vi "SSL Detection Frame Simple Estimator Cameras VelCmd.vi"(0 "Side":enum16{"Esquerdo", "Direito"}(ring)=enum."Direito" caption="Enum", 1 "cameras array":dbl[](array[numeric]), 4 "max ball vel":dbl, 5 "Estimador":T6=enum."Nenhum", 6 "Team":enum16{"Azul", "Amarelo"}(ring) caption="Enum", 7 "Enable":bool=TRUE, 8 "Fps":dbl=40.0, 9 "grSim?":bool, 10 "Field":T1, 11 "Detection Frame":T2 {"robots_blue"."height" format="%+4.3f"; "robots_blue"."pixel_y" format="%+4.3f"; "robots_blue"."pixel_x" format="%+4.3f"; "robots_blue"."orientation" format="%+4.3f"; "robots_blue"."y" format="%+4.3f"; "robots_blue"."confidence" format="%4.3f"; "robots_blue"."x" format="%+4.3f"; "robots_yellow"."height" format="%+4.3f"; "robots_yellow"."pixel_y" format="%+4.3f"; "robots_yellow"."pixel_x" format="%+4.3f"; "robots_yellow"."orientation" format="%+4.3f"; "robots_yellow"."y" format="%+4.3f"; "robots_yellow"."confidence" format="%4.3f"; "robots_yellow"."x" format="%+4.3f"}) -> (2 "Field":T1, 3 "Detection Frame Out":T2 {"robots_blue"."height" format="%+4.3f"; "robots_blue"."pixel_y" format="%+4.3f"; "robots_blue"."pixel_x" format="%+4.3f"; "robots_blue"."orientation" format="%+4.3f"; "robots_blue"."y" format="%+4.3f"; "robots_blue"."confidence" format="%4.3f"; "robots_blue"."x" format="%+4.3f"; "robots_yellow"."height" format="%+4.3f"; "robots_yellow"."pixel_y" format="%+4.3f"; "robots_yellow"."pixel_x" format="%+4.3f"; "robots_yellow"."orientation" format="%+4.3f"; "robots_yellow"."y" format="%+4.3f"; "robots_yellow"."confidence" format="%4.3f"; "robots_yellow"."x" format="%+4.3f"})   [LabVIEW 2020]
uses:
  Controls/SSL Detection Frame.ctl
  Controls/SSL Detection Robot.ctl
  <vilib>/Analysis/Matrix/Datatypes/RealMatrix.ctl
  Controls/SSL Detection Ball.ctl
  Controls/Estimadores.ctl
  <vilib>/Analysis/Matrix/Numeric/Conversions/Array To Matrix - RA.vi
  <vilib>/Analysis/Matrix/NI_Matrix.lvlib
  <vilib>/ptbypt/NI_PtbyPt.lvlib
  Robot_class/FieldFIRASim.ctl
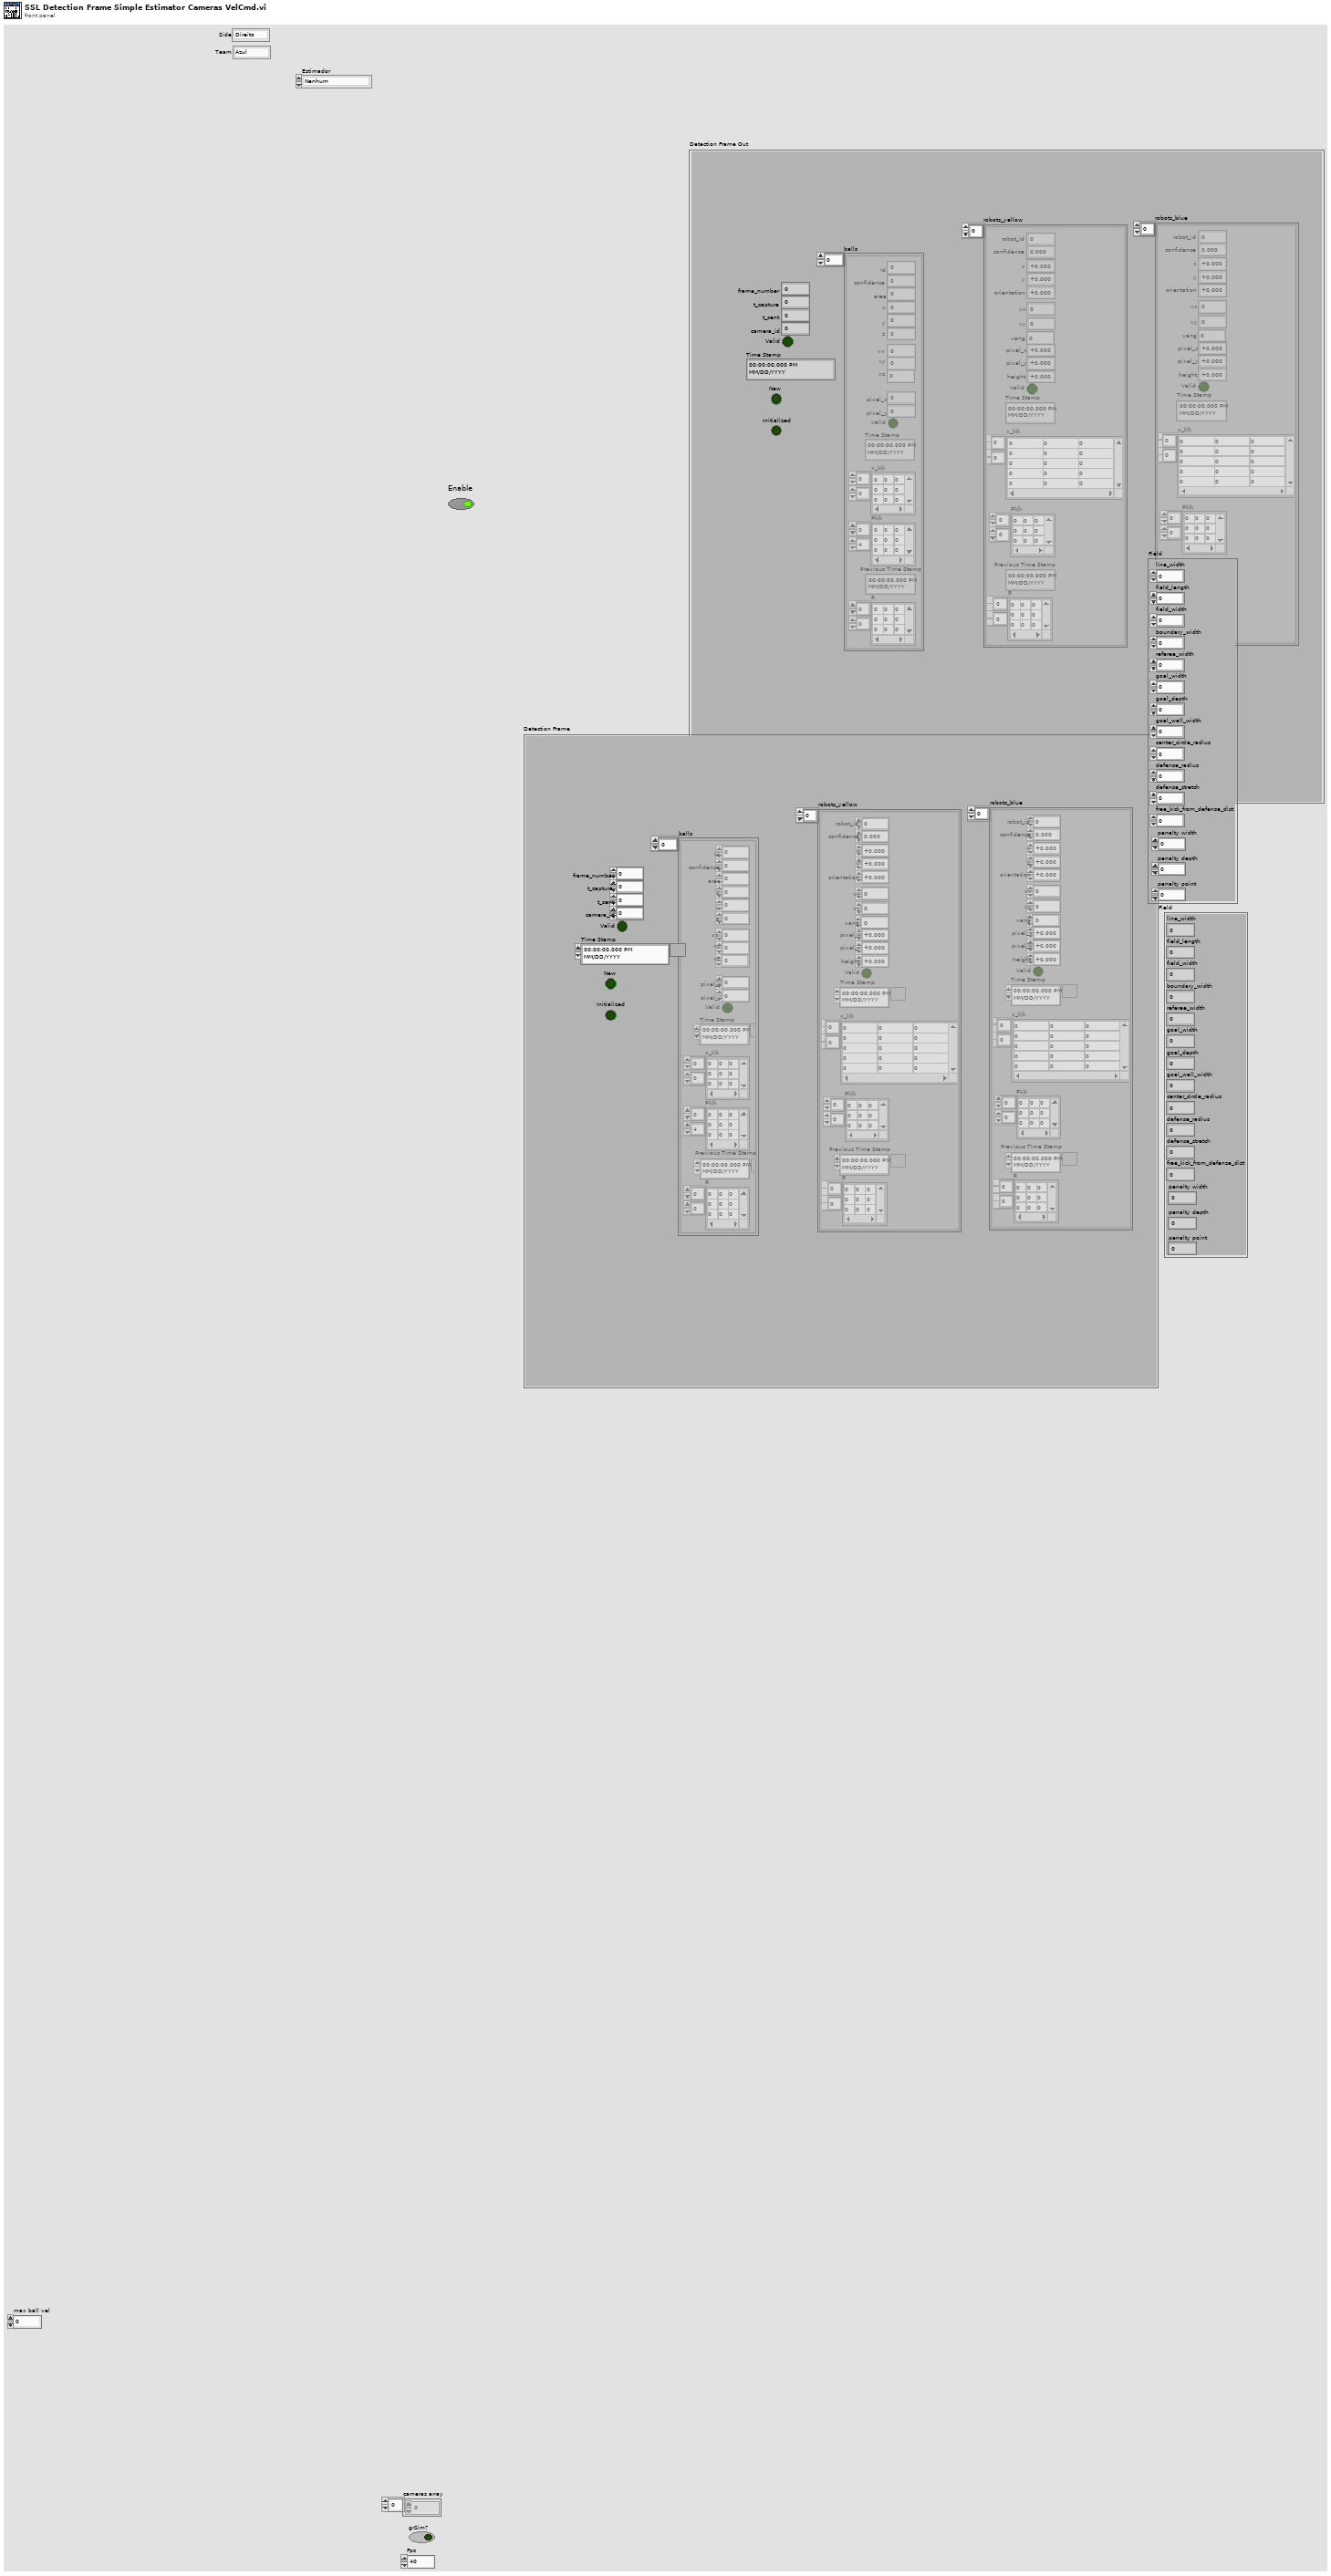
[diagram p1: front panel]
types:
  T1 = typedef "FieldFIRASim.ctl" = cluster{"line_width":u32, "field_length":u32, "field_width":u32, "boundary_width":u32, "referee_width":u32, "goal_width":u32, "goal_depth":u32, "goal_wall_width":u32, "center_circle_radius":u32, "defense_radius":u32, "defense_stretch":u32, "free_kick_from_defense_dist":u32, "penalty width":dbl, "penalty depth":dbl, "penalty point":dbl}
  T2 = typedef "SSL Detection Frame.ctl" = cluster{"frame_number":u32, "t_capture":dbl, "t_sent":dbl, "camera_id":u32, "robots_yellow":T3[], "robots_blue":T3[], "balls":T5[], "Valid":bool, "Time Stamp":timestamp, "New":bool, "Initialized":bool}
  T3 = typedef "SSL Detection Robot.ctl" = cluster{"x":sgl, "robot_id":u32, "confidence":sgl, "y":sgl, "orientation":sgl, "pixel_x":sgl, "pixel_y":sgl, "height":sgl, "Valid":bool, "Time Stamp":timestamp, "x_k|k":T4, "Pk|k":T4, "Previous Time Stamp":timestamp, "R":T4, "vx":dbl, "vy":dbl, "vang":dbl}
  T4 = typedef "NI_Matrix.lvlib/RealMatrix.ctl" = dbl[][]
  T5 = typedef "SSL Detection Ball.ctl" = cluster{"x":sgl, "area":u32, "confidence":sgl, "y":sgl, "z":sgl, "pixel_x":sgl, "pixel_y":sgl, "Valid":bool, "Time Stamp":timestamp, "x_k|k":T4, "Pk|k":T4, "Id":u32, "Previous Time Stamp":timestamp, "R":T4, " vx":sgl, "vy":dbl, "vz":dbl}
  T6 = typedef "Estimadores.ctl" = enum16{"4thDerivate", "2ndDerivate", "Nenhum", "Simples", "Kalman"}
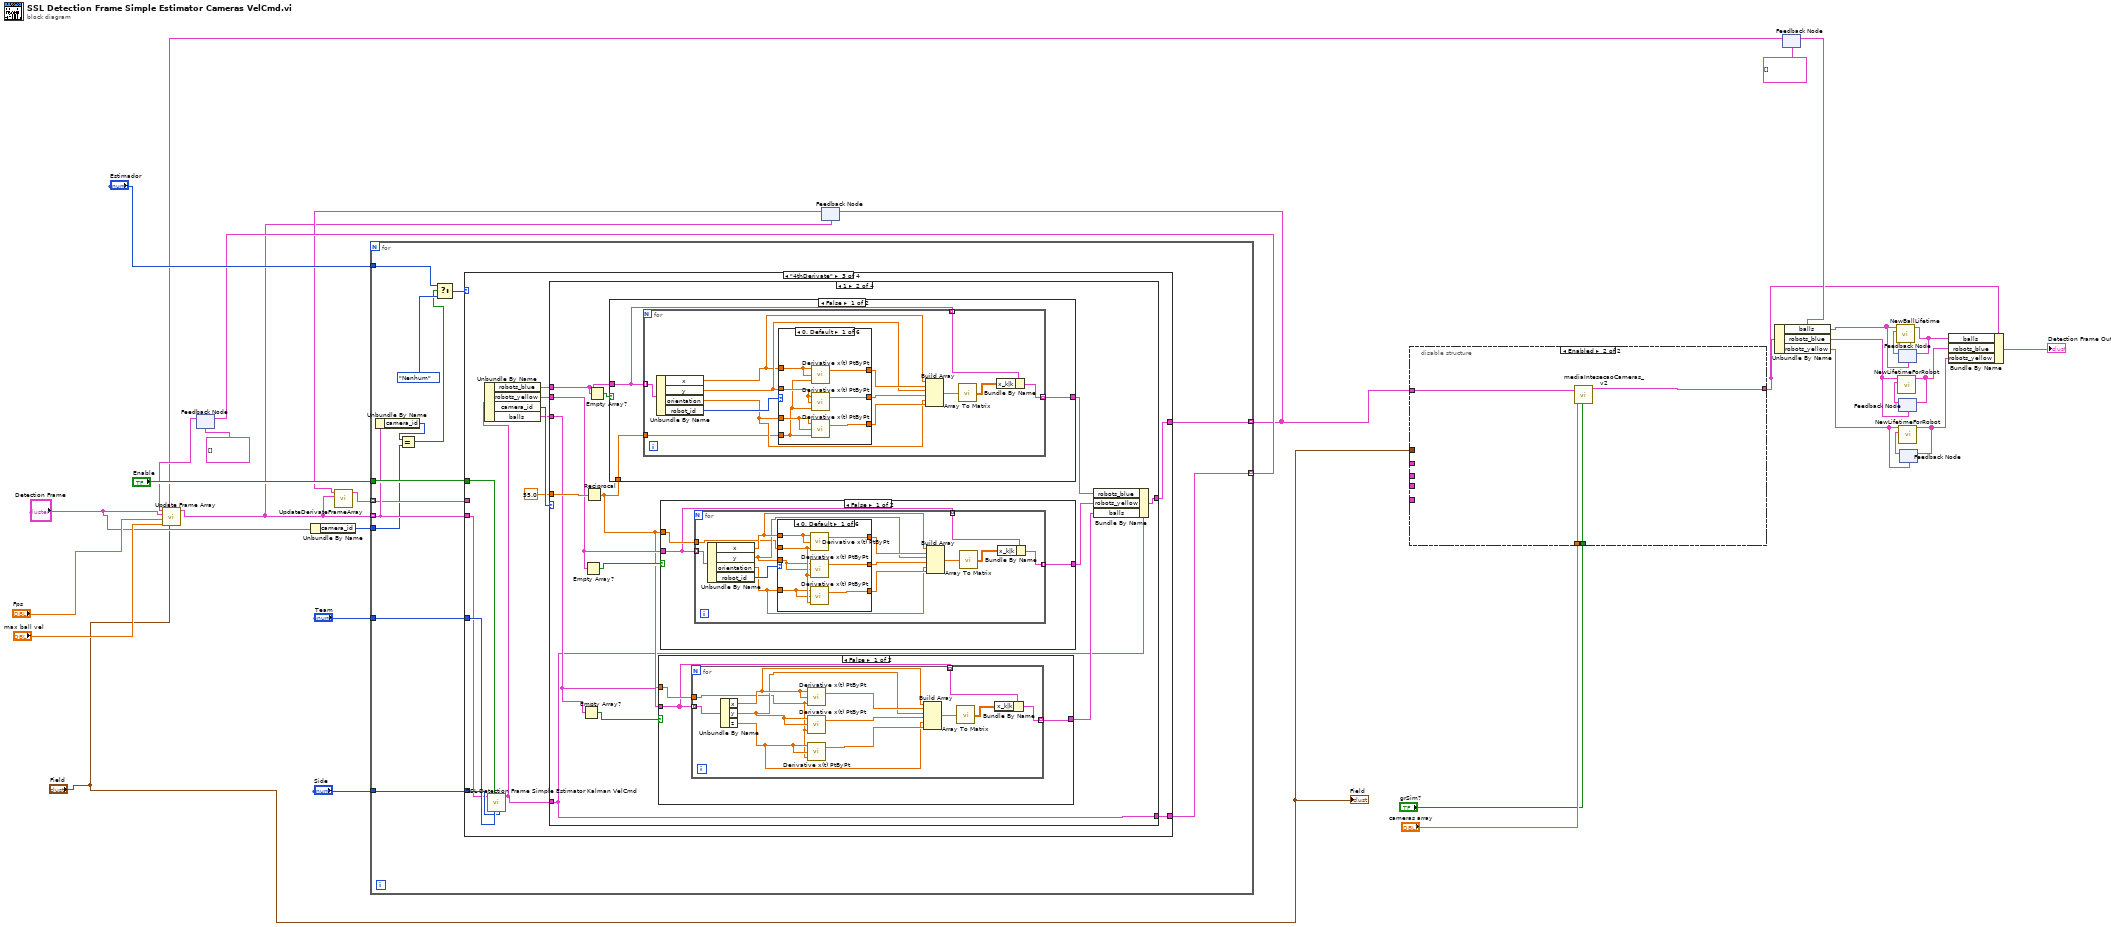
[diagram p0: block diagram]
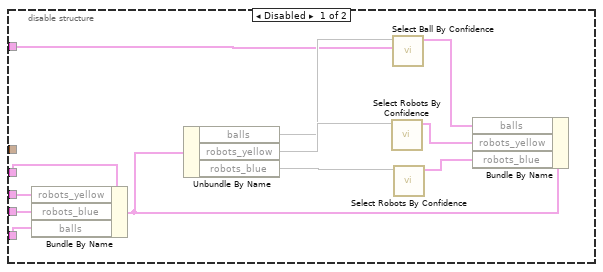
[diagram p2: hidden frame]
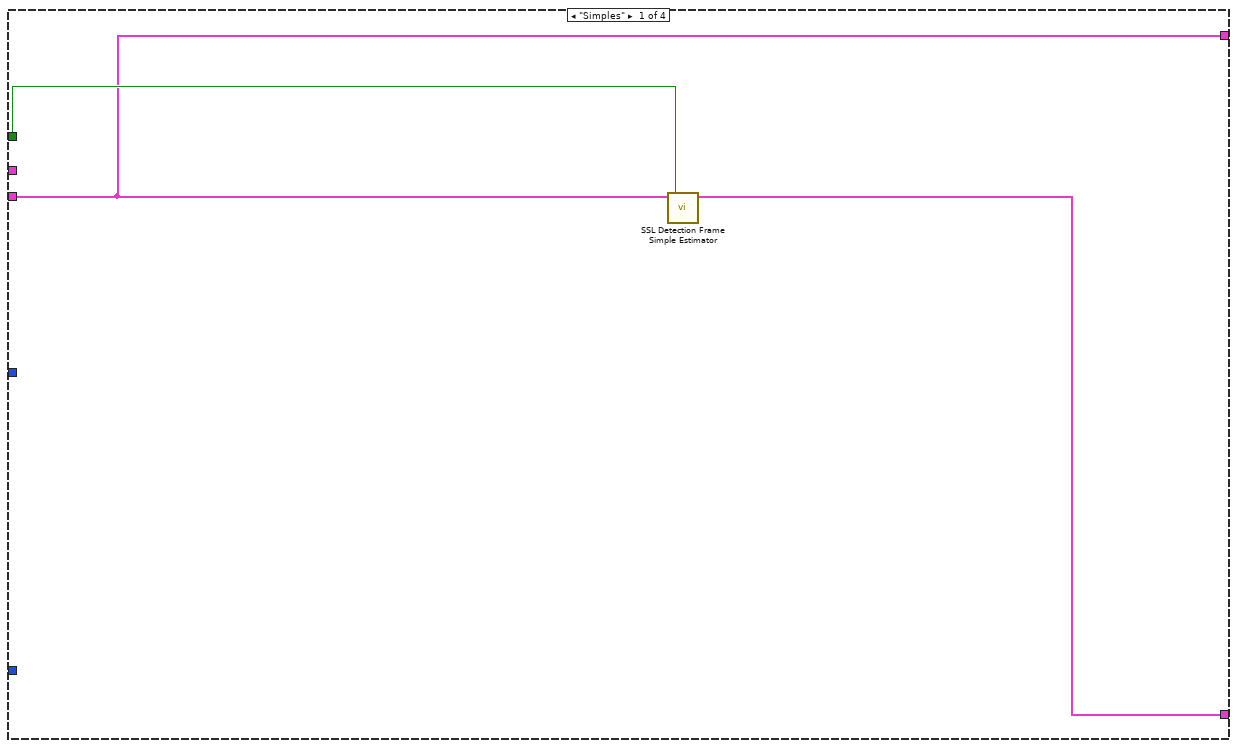
[diagram p3: hidden frame]
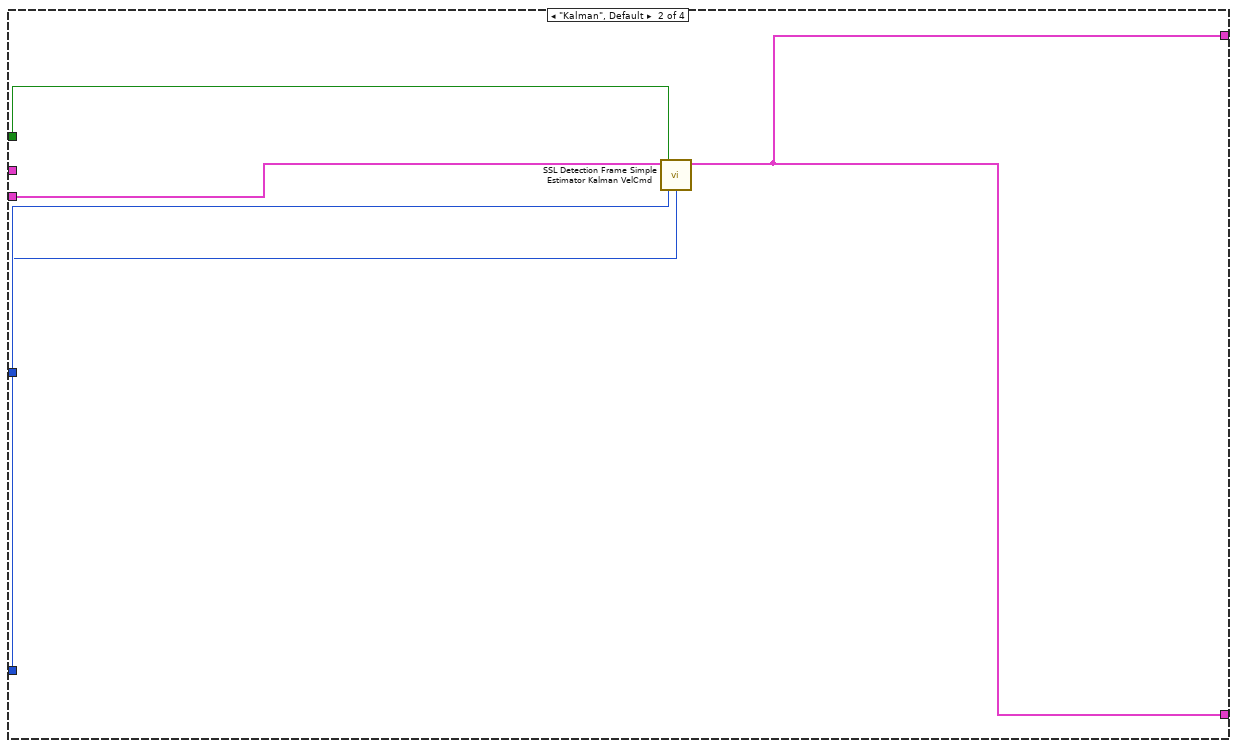
[diagram p4: hidden frame]
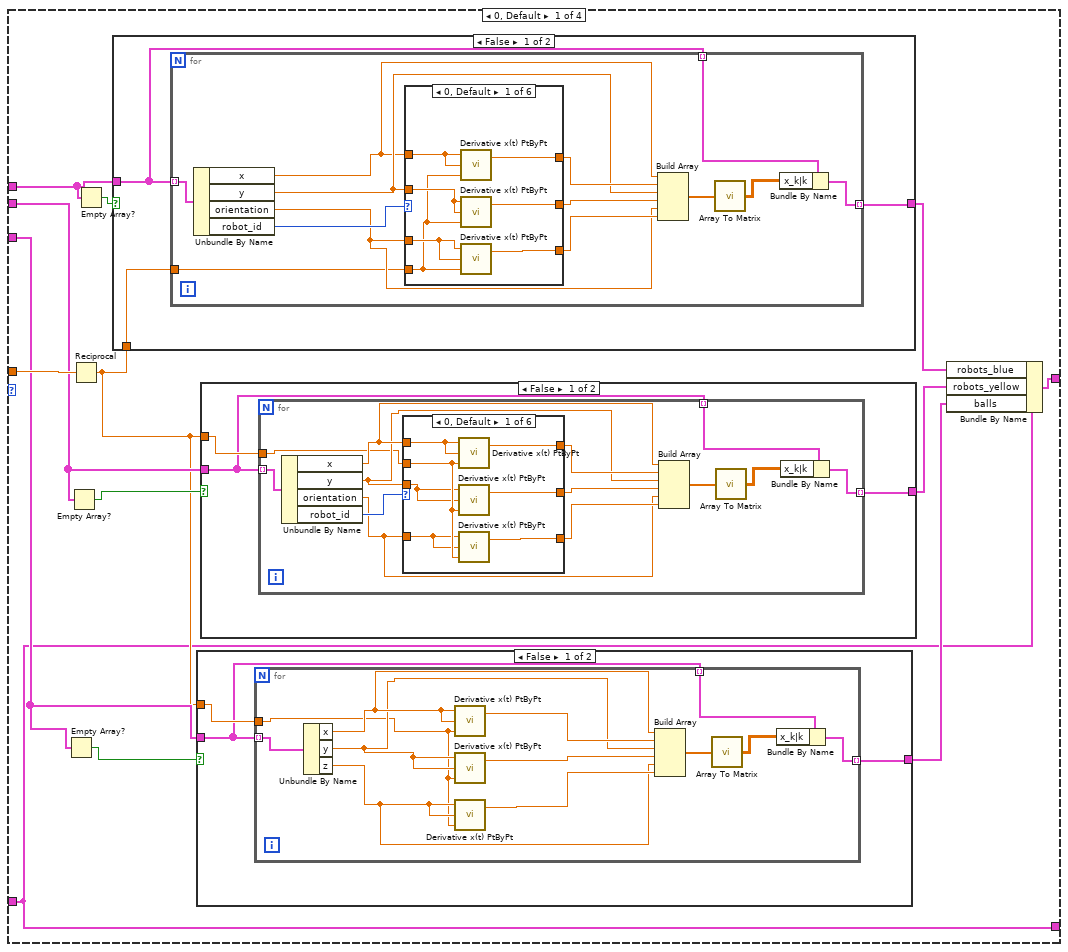
[diagram p5: hidden frame]
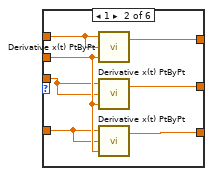
[diagram p7: hidden frame]
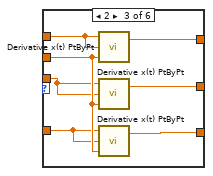
[diagram p8: hidden frame]
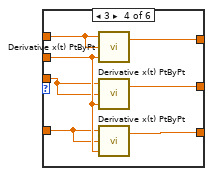
[diagram p9: hidden frame]
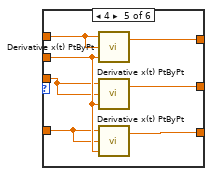
[diagram p10: hidden frame]
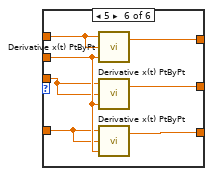
[diagram p11: hidden frame]
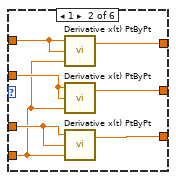
[diagram p13: hidden frame]
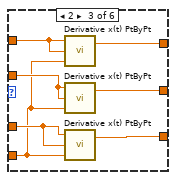
[diagram p14: hidden frame]
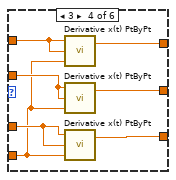
[diagram p15: hidden frame]
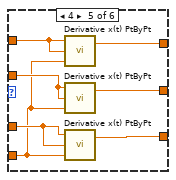
[diagram p16: hidden frame]
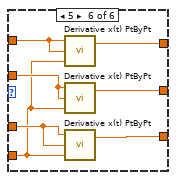
[diagram p17: hidden frame]
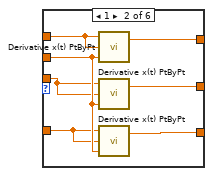
[diagram p20: hidden frame]
diagram:
  n1 = feedback #1(T2[] []) -> (w28:T2[])
  n2 = Unbundle By Name("Detection Frame") -> ("camera_id"=w13:u32)
  n3 = feedback #2(T5[] [] ("balls")) -> (w22:T5[])
  n4 = call "Update Frame Array.vi"("Field"="Field", "balls"=w22, "max ball vel"="max ball vel", "Fps"="Fps", "Detection Frame In"="Detection Frame", "Array Detection Frame In"=w28) -> ("Detection Frame out"=w17:T2[])  [unwired: 4 in, 1 out]
  n5 = feedback #3(w17) -> (w18:T2[])
  n6 = call "UpdateDerivateFrameArray.vi"("Current Detection Frame In"=w17, "Last Array Detection Frame In"=w18) -> ("Sorted Cameras Array"=w16:T2[])  [unwired: 9 in]
  n7 = for {
    tunnel: [w43] -> w26 mode=indexing
    tunnel: "Estimador" -> [w39]
    tunnel: "Enable" -> [w44]
    tunnel: w17 -> [w36] mode=indexing
    tunnel: "Team" -> [w42]
    tunnel: "Side" -> [w41]
    tunnel: [w37] -> w15 mode=indexing
    tunnel: w16 -> [w35] mode=indexing
    tunnel: w13 -> [w33]
    n8 = Unbundle By Name(w36) -> ("camera_id"=w34:u32)
    n9 = Equal?(x=w34, y=w33) -> (x = y?=w32:bool)
    n10 = Select(t=w39, s=w32, f=Estimadores."Nenhum" ("t")) -> (s? t:f=w38:T6)
    n11 = case shown="\"4thDerivate\"" w38 {
      tunnel: [w46 w48 w58 w654] -> w43
      tunnel: w36 -> [w45 w49 w54 w654]
      tunnel: w44 -> [w47 w52 w64 _]
      tunnel: w42 -> [_ w51 w63 _]
      tunnel: w41 -> [_ w50 w62 _]
      tunnel: [w45 w48 w59 w653] -> w37
      tunnel: w35 -> [_ _ _ w653]
      frame "Simples" {
        n12 = call "SSL Detection Frame Simple Estimator.vi"("Enable"=w47, "Detection Frame In"=w45) -> ("Detection Frame Out"=w46:T2)  [unwired: 8 in, 1 out]
      }
      frame "Kalman", Default {
        n13 = call "SSL Detection Frame Simple Estimator Kalman VelCmd.vi"("Lado"=w50, "Time"=w51, "Enable"=w52, "Detection Frame In"=w49) -> ("Detection Frame Out"=w48:T2)  [unwired: 6 in, 1 out]
      }
      frame "4thDerivate" {
        n14 = call "SSL Detection Frame Simple Estimator Kalman VelCmd.vi"("Lado"=w62, "Time"=w63, "Enable"=w64, "Detection Frame In"=w54) -> ("Detection Frame Out"=w53:T2)  [unwired: 6 in, 1 out]
        n15 = Unbundle By Name(w53) -> ("robots_blue"=w61:T3[], "robots_yellow"=w60:T3[], "camera_id"=w57:u32, "balls"=w56:T5[])
        n16 = case shown="1" w57 {
          tunnel: w61 -> [w76 w223 w370 w517]
          tunnel: 55.0 -> [w75 w222 w369 w516]
          tunnel: w60 -> [w73 w220 w367 w514]
          tunnel: [w70 w217 w364 w511] -> w59
          tunnel: [w65 w212 w359 w506] -> w58
          tunnel: w53 -> [w65 w212 w359 w506]
          tunnel: w56 -> [w68 w215 w362 w509]
          frame 0, Default {
            n17 = Empty Array?(array=w68) -> (empty?=w69:bool)
            n18 = Empty Array?(array=w73) -> (empty?=w74:bool)
            n19 = Reciprocal(x=w75) -> (1/x=w67:dbl)
            n20 = Empty Array?(array=w76) -> (empty?=w77:bool)
            n21 = case shown="False" w77 {
              tunnel: w76 -> [w154 w211]
              tunnel: w67 -> [w155 _]
              tunnel: [w153 w211] -> w72
              frame False {
                n22 = for {
                  tunnel: w154 -> [w168] mode=indexing
                  tunnel: w155 -> [w158]
                  tunnel: w154 -> [w166] mode=indexing
                  tunnel: [w157] -> w153 mode=indexing
                  n23 = Unbundle By Name(w168) -> ("x"=w156:sgl, "y"=w160:sgl, "orientation"=w159:sgl, "robot_id"=w167:u32)
                  n24 = case shown="0, Default" w167 {
                    tunnel: w156 -> [w169 w179 w186 w193 w200 w207]
                    tunnel: [w175 w182 w189 w196 w203 w210] -> w165
                    tunnel: [w174 w181 w188 w195 w202 w209] -> w164
                    tunnel: [w173 w180 w187 w194 w201 w208] -> w163
                    tunnel: w160 -> [w172 w178 w185 w192 w199 w206]
                    tunnel: w159 -> [w171 w177 w184 w191 w198 w205]
                    tunnel: w158 -> [w170 w176 w183 w190 w197 w204]
                    frame 0, Default {
                      n25 = call <vilib>:"Derivative x(t) PtByPt.vi"("dt"=w170, "initial condition"=w169, "x"=w169) -> ("dx/dt"=w175:dbl)  [unwired: 1 in, 1 out]
                      n26 = call <vilib>:"Derivative x(t) PtByPt.vi"("dt"=w170, "initial condition"=w172, "x"=w172) -> ("dx/dt"=w174:dbl)  [unwired: 1 in, 1 out]
                      n27 = call <vilib>:"Derivative x(t) PtByPt.vi"("dt"=w170, "initial condition"=w171, "x"=w171) -> ("dx/dt"=w173:dbl)  [unwired: 1 in, 1 out]
                    }
                    frame 1 {
                      n28 = call <vilib>:"Derivative x(t) PtByPt.vi"("dt"=w176, "initial condition"=w179, "x"=w179) -> ("dx/dt"=w182:dbl)  [unwired: 1 in, 1 out]
                      n29 = call <vilib>:"Derivative x(t) PtByPt.vi"("dt"=w176, "initial condition"=w178, "x"=w178) -> ("dx/dt"=w181:dbl)  [unwired: 1 in, 1 out]
                      n30 = call <vilib>:"Derivative x(t) PtByPt.vi"("dt"=w176, "initial condition"=w177, "x"=w177) -> ("dx/dt"=w180:dbl)  [unwired: 1 in, 1 out]
                    }
                    frame 2 {
                      n31 = call <vilib>:"Derivative x(t) PtByPt.vi"("dt"=w183, "initial condition"=w186, "x"=w186) -> ("dx/dt"=w189:dbl)  [unwired: 1 in, 1 out]
                      n32 = call <vilib>:"Derivative x(t) PtByPt.vi"("dt"=w183, "initial condition"=w185, "x"=w185) -> ("dx/dt"=w188:dbl)  [unwired: 1 in, 1 out]
                      n33 = call <vilib>:"Derivative x(t) PtByPt.vi"("dt"=w183, "initial condition"=w184, "x"=w184) -> ("dx/dt"=w187:dbl)  [unwired: 1 in, 1 out]
                    }
                    frame 3 {
                      n34 = call <vilib>:"Derivative x(t) PtByPt.vi"("dt"=w190, "initial condition"=w193, "x"=w193) -> ("dx/dt"=w196:dbl)  [unwired: 1 in, 1 out]
                      n35 = call <vilib>:"Derivative x(t) PtByPt.vi"("dt"=w190, "initial condition"=w192, "x"=w192) -> ("dx/dt"=w195:dbl)  [unwired: 1 in, 1 out]
                      n36 = call <vilib>:"Derivative x(t) PtByPt.vi"("dt"=w190, "initial condition"=w191, "x"=w191) -> ("dx/dt"=w194:dbl)  [unwired: 1 in, 1 out]
                    }
                    frame 4 {
                      n37 = call <vilib>:"Derivative x(t) PtByPt.vi"("dt"=w197, "initial condition"=w200, "x"=w200) -> ("dx/dt"=w203:dbl)  [unwired: 1 in, 1 out]
                      n38 = call <vilib>:"Derivative x(t) PtByPt.vi"("dt"=w197, "initial condition"=w199, "x"=w199) -> ("dx/dt"=w202:dbl)  [unwired: 1 in, 1 out]
                      n39 = call <vilib>:"Derivative x(t) PtByPt.vi"("dt"=w197, "initial condition"=w198, "x"=w198) -> ("dx/dt"=w201:dbl)  [unwired: 1 in, 1 out]
                    }
                    frame 5 {
                      n40 = call <vilib>:"Derivative x(t) PtByPt.vi"("dt"=w204, "initial condition"=w207, "x"=w207) -> ("dx/dt"=w210:dbl)  [unwired: 1 in, 1 out]
                      n41 = call <vilib>:"Derivative x(t) PtByPt.vi"("dt"=w204, "initial condition"=w206, "x"=w206) -> ("dx/dt"=w209:dbl)  [unwired: 1 in, 1 out]
                      n42 = call <vilib>:"Derivative x(t) PtByPt.vi"("dt"=w204, "initial condition"=w205, "x"=w205) -> ("dx/dt"=w208:dbl)  [unwired: 1 in, 1 out]
                    }
                  }
                  n43 = Build Array(w156, w165, w160, w164, w159, w163) -> (w162:dbl[])
                  n44 = call-poly <vilib>:"Array To Matrix.vi"("Real 1D Array"=w162) -> ("Real Matrix (Column Vector)"=w161:T4)
                  n45 = Bundle By Name(cluster=w166, "x_k|k"=w161) -> (w157:T3)
                }
              }
              frame True {
              }
            }
            n46 = case shown="False" w69 {
              tunnel: w68 -> [w79 w93]
              tunnel: w67 -> [w80 _]
              tunnel: [w78 w93] -> w66
              frame False {
                n47 = for {
                  tunnel: w79 -> [w92] mode=indexing
                  tunnel: w80 -> [w81]
                  tunnel: w79 -> [w91] mode=indexing
                  tunnel: [w82] -> w78 mode=indexing
                  n48 = Unbundle By Name(w92) -> ("x"=w86:sgl, "y"=w85:sgl, "z"=w87:sgl)
                  n49 = call <vilib>:"Derivative x(t) PtByPt.vi"("dt"=w81, "initial condition"=w86, "x"=w86) -> ("dx/dt"=w90:dbl)  [unwired: 1 in, 1 out]
                  n50 = call <vilib>:"Derivative x(t) PtByPt.vi"("dt"=w81, "initial condition"=w85, "x"=w85) -> ("dx/dt"=w89:dbl)  [unwired: 1 in, 1 out]
                  n51 = call <vilib>:"Derivative x(t) PtByPt.vi"("dt"=w81, "initial condition"=w87, "x"=w87) -> ("dx/dt"=w88:dbl)  [unwired: 1 in, 1 out]
                  n52 = Build Array(w86, w90, w85, w89, w87, w88) -> (w84:dbl[])
                  n53 = call-poly <vilib>:"Array To Matrix.vi"("Real 1D Array"=w84) -> ("Real Matrix (Column Vector)"=w83:T4)
                  n54 = Bundle By Name(cluster=w91, "x_k|k"=w83) -> (w82:T5)
                }
              }
              frame True {
              }
            }
            n55 = case shown="False" w74 {
              tunnel: w73 -> [w95 w152]
              tunnel: w67 -> [w96 _]
              tunnel: [w94 w152] -> w71
              frame False {
                n56 = for {
                  tunnel: w95 -> [w109] mode=indexing
                  tunnel: w96 -> [w97]
                  tunnel: w95 -> [w107] mode=indexing
                  tunnel: [w98] -> w94 mode=indexing
                  n57 = Unbundle By Name(w109) -> ("x"=w102:sgl, "y"=w101:sgl, "orientation"=w103:sgl, "robot_id"=w108:u32)
                  n58 = case shown="0, Default" w108 {
                    tunnel: w102 -> [w113 w120 w127 w134 w141 w148]
                    tunnel: w101 -> [w111 w118 w125 w132 w139 w146]
                    tunnel: w103 -> [w110 w117 w124 w131 w138 w145]
                    tunnel: [w116 w123 w130 w137 w144 w151] -> w106
                    tunnel: [w115 w122 w129 w136 w143 w150] -> w105
                    tunnel: [w114 w121 w128 w135 w142 w149] -> w104
                    tunnel: w97 -> [w112 w119 w126 w133 w140 w147]
                    frame 0, Default {
                      n59 = call <vilib>:"Derivative x(t) PtByPt.vi"("dt"=w112, "initial condition"=w113, "x"=w113) -> ("dx/dt"=w116:dbl)  [unwired: 1 in, 1 out]
                      n60 = call <vilib>:"Derivative x(t) PtByPt.vi"("dt"=w112, "initial condition"=w111, "x"=w111) -> ("dx/dt"=w115:dbl)  [unwired: 1 in, 1 out]
                      n61 = call <vilib>:"Derivative x(t) PtByPt.vi"("dt"=w112, "initial condition"=w110, "x"=w110) -> ("dx/dt"=w114:dbl)  [unwired: 1 in, 1 out]
                    }
                    frame 1 {
                      n62 = call <vilib>:"Derivative x(t) PtByPt.vi"("dt"=w119, "initial condition"=w120, "x"=w120) -> ("dx/dt"=w123:dbl)  [unwired: 1 in, 1 out]
                      n63 = call <vilib>:"Derivative x(t) PtByPt.vi"("dt"=w119, "initial condition"=w118, "x"=w118) -> ("dx/dt"=w122:dbl)  [unwired: 1 in, 1 out]
                      n64 = call <vilib>:"Derivative x(t) PtByPt.vi"("dt"=w119, "initial condition"=w117, "x"=w117) -> ("dx/dt"=w121:dbl)  [unwired: 1 in, 1 out]
                    }
                    frame 2 {
                      n65 = call <vilib>:"Derivative x(t) PtByPt.vi"("dt"=w126, "initial condition"=w127, "x"=w127) -> ("dx/dt"=w130:dbl)  [unwired: 1 in, 1 out]
                      n66 = call <vilib>:"Derivative x(t) PtByPt.vi"("dt"=w126, "initial condition"=w125, "x"=w125) -> ("dx/dt"=w129:dbl)  [unwired: 1 in, 1 out]
                      n67 = call <vilib>:"Derivative x(t) PtByPt.vi"("dt"=w126, "initial condition"=w124, "x"=w124) -> ("dx/dt"=w128:dbl)  [unwired: 1 in, 1 out]
                    }
                    frame 3 {
                      n68 = call <vilib>:"Derivative x(t) PtByPt.vi"("dt"=w133, "initial condition"=w134, "x"=w134) -> ("dx/dt"=w137:dbl)  [unwired: 1 in, 1 out]
                      n69 = call <vilib>:"Derivative x(t) PtByPt.vi"("dt"=w133, "initial condition"=w132, "x"=w132) -> ("dx/dt"=w136:dbl)  [unwired: 1 in, 1 out]
                      n70 = call <vilib>:"Derivative x(t) PtByPt.vi"("dt"=w133, "initial condition"=w131, "x"=w131) -> ("dx/dt"=w135:dbl)  [unwired: 1 in, 1 out]
                    }
                    frame 4 {
                      n71 = call <vilib>:"Derivative x(t) PtByPt.vi"("dt"=w140, "initial condition"=w141, "x"=w141) -> ("dx/dt"=w144:dbl)  [unwired: 1 in, 1 out]
                      n72 = call <vilib>:"Derivative x(t) PtByPt.vi"("dt"=w140, "initial condition"=w139, "x"=w139) -> ("dx/dt"=w143:dbl)  [unwired: 1 in, 1 out]
                      n73 = call <vilib>:"Derivative x(t) PtByPt.vi"("dt"=w140, "initial condition"=w138, "x"=w138) -> ("dx/dt"=w142:dbl)  [unwired: 1 in, 1 out]
                    }
                    frame 5 {
                      n74 = call <vilib>:"Derivative x(t) PtByPt.vi"("dt"=w147, "initial condition"=w148, "x"=w148) -> ("dx/dt"=w151:dbl)  [unwired: 1 in, 1 out]
                      n75 = call <vilib>:"Derivative x(t) PtByPt.vi"("dt"=w147, "initial condition"=w146, "x"=w146) -> ("dx/dt"=w150:dbl)  [unwired: 1 in, 1 out]
                      n76 = call <vilib>:"Derivative x(t) PtByPt.vi"("dt"=w147, "initial condition"=w145, "x"=w145) -> ("dx/dt"=w149:dbl)  [unwired: 1 in, 1 out]
                    }
                  }
                  n77 = Build Array(w102, w106, w101, w105, w103, w104) -> (w100:dbl[])
                  n78 = call-poly <vilib>:"Array To Matrix.vi"("Real 1D Array"=w100) -> ("Real Matrix (Column Vector)"=w99:T4)
                  n79 = Bundle By Name(cluster=w107, "x_k|k"=w99) -> (w98:T3)
                }
              }
              frame True {
              }
            }
            n80 = Bundle By Name(cluster=w65, "robots_blue"=w72, "robots_yellow"=w71, "balls"=w66) -> (w70:T2)
          }
          frame 1 {
            n81 = Empty Array?(array=w215) -> (empty?=w216:bool)
            n82 = Empty Array?(array=w220) -> (empty?=w221:bool)
            n83 = Reciprocal(x=w222) -> (1/x=w214:dbl)
            n84 = Empty Array?(array=w223) -> (empty?=w224:bool)
            n85 = case shown="False" w224 {
              tunnel: w223 -> [w301 w358]
              tunnel: w214 -> [w302 _]
              tunnel: [w300 w358] -> w219
              frame False {
                n86 = for {
                  tunnel: w301 -> [w315] mode=indexing
                  tunnel: w302 -> [w305]
                  tunnel: w301 -> [w313] mode=indexing
                  tunnel: [w304] -> w300 mode=indexing
                  n87 = Unbundle By Name(w315) -> ("x"=w303:sgl, "y"=w307:sgl, "orientation"=w306:sgl, "robot_id"=w314:u32)
                  n88 = case shown="0, Default" w314 {
                    tunnel: w303 -> [w316 w326 w333 w340 w347 w354]
                    tunnel: [w322 w329 w336 w343 w350 w357] -> w312
                    tunnel: [w321 w328 w335 w342 w349 w356] -> w311
                    tunnel: [w320 w327 w334 w341 w348 w355] -> w310
                    tunnel: w307 -> [w319 w325 w332 w339 w346 w353]
                    tunnel: w306 -> [w318 w324 w331 w338 w345 w352]
                    tunnel: w305 -> [w317 w323 w330 w337 w344 w351]
                    frame 0, Default {
                      n89 = call <vilib>:"Derivative x(t) PtByPt.vi"("dt"=w317, "initial condition"=w316, "x"=w316) -> ("dx/dt"=w322:dbl)  [unwired: 1 in, 1 out]
                      n90 = call <vilib>:"Derivative x(t) PtByPt.vi"("dt"=w317, "initial condition"=w319, "x"=w319) -> ("dx/dt"=w321:dbl)  [unwired: 1 in, 1 out]
                      n91 = call <vilib>:"Derivative x(t) PtByPt.vi"("dt"=w317, "initial condition"=w318, "x"=w318) -> ("dx/dt"=w320:dbl)  [unwired: 1 in, 1 out]
                    }
                    frame 1 {
                      n92 = call <vilib>:"Derivative x(t) PtByPt.vi"("dt"=w323, "initial condition"=w326, "x"=w326) -> ("dx/dt"=w329:dbl)  [unwired: 1 in, 1 out]
                      n93 = call <vilib>:"Derivative x(t) PtByPt.vi"("dt"=w323, "initial condition"=w325, "x"=w325) -> ("dx/dt"=w328:dbl)  [unwired: 1 in, 1 out]
                      n94 = call <vilib>:"Derivative x(t) PtByPt.vi"("dt"=w323, "initial condition"=w324, "x"=w324) -> ("dx/dt"=w327:dbl)  [unwired: 1 in, 1 out]
                    }
                    frame 2 {
                      n95 = call <vilib>:"Derivative x(t) PtByPt.vi"("dt"=w330, "initial condition"=w333, "x"=w333) -> ("dx/dt"=w336:dbl)  [unwired: 1 in, 1 out]
                      n96 = call <vilib>:"Derivative x(t) PtByPt.vi"("dt"=w330, "initial condition"=w332, "x"=w332) -> ("dx/dt"=w335:dbl)  [unwired: 1 in, 1 out]
                      n97 = call <vilib>:"Derivative x(t) PtByPt.vi"("dt"=w330, "initial condition"=w331, "x"=w331) -> ("dx/dt"=w334:dbl)  [unwired: 1 in, 1 out]
                    }
                    frame 3 {
                      n98 = call <vilib>:"Derivative x(t) PtByPt.vi"("dt"=w337, "initial condition"=w340, "x"=w340) -> ("dx/dt"=w343:dbl)  [unwired: 1 in, 1 out]
                      n99 = call <vilib>:"Derivative x(t) PtByPt.vi"("dt"=w337, "initial condition"=w339, "x"=w339) -> ("dx/dt"=w342:dbl)  [unwired: 1 in, 1 out]
                      n100 = call <vilib>:"Derivative x(t) PtByPt.vi"("dt"=w337, "initial condition"=w338, "x"=w338) -> ("dx/dt"=w341:dbl)  [unwired: 1 in, 1 out]
                    }
                    frame 4 {
                      n101 = call <vilib>:"Derivative x(t) PtByPt.vi"("dt"=w344, "initial condition"=w347, "x"=w347) -> ("dx/dt"=w350:dbl)  [unwired: 1 in, 1 out]
                      n102 = call <vilib>:"Derivative x(t) PtByPt.vi"("dt"=w344, "initial condition"=w346, "x"=w346) -> ("dx/dt"=w349:dbl)  [unwired: 1 in, 1 out]
                      n103 = call <vilib>:"Derivative x(t) PtByPt.vi"("dt"=w344, "initial condition"=w345, "x"=w345) -> ("dx/dt"=w348:dbl)  [unwired: 1 in, 1 out]
                    }
                    frame 5 {
                      n104 = call <vilib>:"Derivative x(t) PtByPt.vi"("dt"=w351, "initial condition"=w354, "x"=w354) -> ("dx/dt"=w357:dbl)  [unwired: 1 in, 1 out]
                      n105 = call <vilib>:"Derivative x(t) PtByPt.vi"("dt"=w351, "initial condition"=w353, "x"=w353) -> ("dx/dt"=w356:dbl)  [unwired: 1 in, 1 out]
                      n106 = call <vilib>:"Derivative x(t) PtByPt.vi"("dt"=w351, "initial condition"=w352, "x"=w352) -> ("dx/dt"=w355:dbl)  [unwired: 1 in, 1 out]
                    }
                  }
                  n107 = Build Array(w303, w312, w307, w311, w306, w310) -> (w309:dbl[])
                  n108 = call-poly <vilib>:"Array To Matrix.vi"("Real 1D Array"=w309) -> ("Real Matrix (Column Vector)"=w308:T4)
                  n109 = Bundle By Name(cluster=w313, "x_k|k"=w308) -> (w304:T3)
                }
              }
              frame True {
              }
            }
            n110 = case shown="False" w216 {
              tunnel: w215 -> [w226 w240]
              tunnel: w214 -> [w227 _]
              tunnel: [w225 w240] -> w213
              frame False {
                n111 = for {
                  tunnel: w226 -> [w239] mode=indexing
                  tunnel: w227 -> [w228]
                  tunnel: w226 -> [w238] mode=indexing
                  tunnel: [w229] -> w225 mode=indexing
                  n112 = Unbundle By Name(w239) -> ("x"=w233:sgl, "y"=w232:sgl, "z"=w234:sgl)
                  n113 = call <vilib>:"Derivative x(t) PtByPt.vi"("dt"=w228, "initial condition"=w233, "x"=w233) -> ("dx/dt"=w237:dbl)  [unwired: 1 in, 1 out]
                  n114 = call <vilib>:"Derivative x(t) PtByPt.vi"("dt"=w228, "initial condition"=w232, "x"=w232) -> ("dx/dt"=w236:dbl)  [unwired: 1 in, 1 out]
                  n115 = call <vilib>:"Derivative x(t) PtByPt.vi"("dt"=w228, "initial condition"=w234, "x"=w234) -> ("dx/dt"=w235:dbl)  [unwired: 1 in, 1 out]
                  n116 = Build Array(w233, w237, w232, w236, w234, w235) -> (w231:dbl[])
                  n117 = call-poly <vilib>:"Array To Matrix.vi"("Real 1D Array"=w231) -> ("Real Matrix (Column Vector)"=w230:T4)
                  n118 = Bundle By Name(cluster=w238, "x_k|k"=w230) -> (w229:T5)
                }
              }
              frame True {
              }
            }
            n119 = case shown="False" w221 {
              tunnel: w220 -> [w242 w299]
              tunnel: w214 -> [w243 _]
              tunnel: [w241 w299] -> w218
              frame False {
                n120 = for {
                  tunnel: w242 -> [w256] mode=indexing
                  tunnel: w243 -> [w244]
                  tunnel: w242 -> [w254] mode=indexing
                  tunnel: [w245] -> w241 mode=indexing
                  n121 = Unbundle By Name(w256) -> ("x"=w249:sgl, "y"=w248:sgl, "orientation"=w250:sgl, "robot_id"=w255:u32)
                  n122 = case shown="0, Default" w255 {
                    tunnel: w249 -> [w260 w267 w274 w281 w288 w295]
                    tunnel: w248 -> [w258 w265 w272 w279 w286 w293]
                    tunnel: w250 -> [w257 w264 w271 w278 w285 w292]
                    tunnel: [w263 w270 w277 w284 w291 w298] -> w253
                    tunnel: [w262 w269 w276 w283 w290 w297] -> w252
                    tunnel: [w261 w268 w275 w282 w289 w296] -> w251
                    tunnel: w244 -> [w259 w266 w273 w280 w287 w294]
                    frame 0, Default {
                      n123 = call <vilib>:"Derivative x(t) PtByPt.vi"("dt"=w259, "initial condition"=w260, "x"=w260) -> ("dx/dt"=w263:dbl)  [unwired: 1 in, 1 out]
                      n124 = call <vilib>:"Derivative x(t) PtByPt.vi"("dt"=w259, "initial condition"=w258, "x"=w258) -> ("dx/dt"=w262:dbl)  [unwired: 1 in, 1 out]
                      n125 = call <vilib>:"Derivative x(t) PtByPt.vi"("dt"=w259, "initial condition"=w257, "x"=w257) -> ("dx/dt"=w261:dbl)  [unwired: 1 in, 1 out]
                    }
                    frame 1 {
                      n126 = call <vilib>:"Derivative x(t) PtByPt.vi"("dt"=w266, "initial condition"=w267, "x"=w267) -> ("dx/dt"=w270:dbl)  [unwired: 1 in, 1 out]
                      n127 = call <vilib>:"Derivative x(t) PtByPt.vi"("dt"=w266, "initial condition"=w265, "x"=w265) -> ("dx/dt"=w269:dbl)  [unwired: 1 in, 1 out]
                      n128 = call <vilib>:"Derivative x(t) PtByPt.vi"("dt"=w266, "initial condition"=w264, "x"=w264) -> ("dx/dt"=w268:dbl)  [unwired: 1 in, 1 out]
                    }
                    frame 2 {
                      n129 = call <vilib>:"Derivative x(t) PtByPt.vi"("dt"=w273, "initial condition"=w274, "x"=w274) -> ("dx/dt"=w277:dbl)  [unwired: 1 in, 1 out]
                      n130 = call <vilib>:"Derivative x(t) PtByPt.vi"("dt"=w273, "initial condition"=w272, "x"=w272) -> ("dx/dt"=w276:dbl)  [unwired: 1 in, 1 out]
                      n131 = call <vilib>:"Derivative x(t) PtByPt.vi"("dt"=w273, "initial condition"=w271, "x"=w271) -> ("dx/dt"=w275:dbl)  [unwired: 1 in, 1 out]
                    }
                    frame 3 {
                      n132 = call <vilib>:"Derivative x(t) PtByPt.vi"("dt"=w280, "initial condition"=w281, "x"=w281) -> ("dx/dt"=w284:dbl)  [unwired: 1 in, 1 out]
                      n133 = call <vilib>:"Derivative x(t) PtByPt.vi"("dt"=w280, "initial condition"=w279, "x"=w279) -> ("dx/dt"=w283:dbl)  [unwired: 1 in, 1 out]
                      n134 = call <vilib>:"Derivative x(t) PtByPt.vi"("dt"=w280, "initial condition"=w278, "x"=w278) -> ("dx/dt"=w282:dbl)  [unwired: 1 in, 1 out]
                    }
                    frame 4 {
                      n135 = call <vilib>:"Derivative x(t) PtByPt.vi"("dt"=w287, "initial condition"=w288, "x"=w288) -> ("dx/dt"=w291:dbl)  [unwired: 1 in, 1 out]
                      n136 = call <vilib>:"Derivative x(t) PtByPt.vi"("dt"=w287, "initial condition"=w286, "x"=w286) -> ("dx/dt"=w290:dbl)  [unwired: 1 in, 1 out]
                      n137 = call <vilib>:"Derivative x(t) PtByPt.vi"("dt"=w287, "initial condition"=w285, "x"=w285) -> ("dx/dt"=w289:dbl)  [unwired: 1 in, 1 out]
                    }
                    frame 5 {
                      n138 = call <vilib>:"Derivative x(t) PtByPt.vi"("dt"=w294, "initial condition"=w295, "x"=w295) -> ("dx/dt"=w298:dbl)  [unwired: 1 in, 1 out]
                      n139 = call <vilib>:"Derivative x(t) PtByPt.vi"("dt"=w294, "initial condition"=w293, "x"=w293) -> ("dx/dt"=w297:dbl)  [unwired: 1 in, 1 out]
                      n140 = call <vilib>:"Derivative x(t) PtByPt.vi"("dt"=w294, "initial condition"=w292, "x"=w292) -> ("dx/dt"=w296:dbl)  [unwired: 1 in, 1 out]
                    }
                  }
                  n141 = Build Array(w249, w253, w248, w252, w250, w251) -> (w247:dbl[])
                  n142 = call-poly <vilib>:"Array To Matrix.vi"("Real 1D Array"=w247) -> ("Real Matrix (Column Vector)"=w246:T4)
                  n143 = Bundle By Name(cluster=w254, "x_k|k"=w246) -> (w245:T3)
                }
              }
              frame True {
              }
            }
            n144 = Bundle By Name(cluster=w212, "robots_blue"=w219, "robots_yellow"=w218, "balls"=w213) -> (w217:T2)
          }
          frame 2 {
            n145 = Empty Array?(array=w362) -> (empty?=w363:bool)
            n146 = Empty Array?(array=w367) -> (empty?=w368:bool)
            n147 = Reciprocal(x=w369) -> (1/x=w361:dbl)
            n148 = Empty Array?(array=w370) -> (empty?=w371:bool)
            n149 = case shown="False" w371 {
              tunnel: w370 -> [w448 w505]
              tunnel: w361 -> [w449 _]
              tunnel: [w447 w505] -> w366
              frame False {
                n150 = for {
                  tunnel: w448 -> [w462] mode=indexing
                  tunnel: w449 -> [w452]
                  tunnel: w448 -> [w460] mode=indexing
                  tunnel: [w451] -> w447 mode=indexing
                  n151 = Unbundle By Name(w462) -> ("x"=w450:sgl, "y"=w454:sgl, "orientation"=w453:sgl, "robot_id"=w461:u32)
                  n152 = case shown="0, Default" w461 {
                    tunnel: w450 -> [w463 w473 w480 w487 w494 w501]
                    tunnel: [w469 w476 w483 w490 w497 w504] -> w459
                    tunnel: [w468 w475 w482 w489 w496 w503] -> w458
                    tunnel: [w467 w474 w481 w488 w495 w502] -> w457
                    tunnel: w454 -> [w466 w472 w479 w486 w493 w500]
                    tunnel: w453 -> [w465 w471 w478 w485 w492 w499]
                    tunnel: w452 -> [w464 w470 w477 w484 w491 w498]
                    frame 0, Default {
                      n153 = call <vilib>:"Derivative x(t) PtByPt.vi"("dt"=w464, "initial condition"=w463, "x"=w463) -> ("dx/dt"=w469:dbl)  [unwired: 1 in, 1 out]
                      n154 = call <vilib>:"Derivative x(t) PtByPt.vi"("dt"=w464, "initial condition"=w466, "x"=w466) -> ("dx/dt"=w468:dbl)  [unwired: 1 in, 1 out]
                      n155 = call <vilib>:"Derivative x(t) PtByPt.vi"("dt"=w464, "initial condition"=w465, "x"=w465) -> ("dx/dt"=w467:dbl)  [unwired: 1 in, 1 out]
                    }
                    frame 1 {
                      n156 = call <vilib>:"Derivative x(t) PtByPt.vi"("dt"=w470, "initial condition"=w473, "x"=w473) -> ("dx/dt"=w476:dbl)  [unwired: 1 in, 1 out]
                      n157 = call <vilib>:"Derivative x(t) PtByPt.vi"("dt"=w470, "initial condition"=w472, "x"=w472) -> ("dx/dt"=w475:dbl)  [unwired: 1 in, 1 out]
                      n158 = call <vilib>:"Derivative x(t) PtByPt.vi"("dt"=w470, "initial condition"=w471, "x"=w471) -> ("dx/dt"=w474:dbl)  [unwired: 1 in, 1 out]
                    }
                    frame 2 {
                      n159 = call <vilib>:"Derivative x(t) PtByPt.vi"("dt"=w477, "initial condition"=w480, "x"=w480) -> ("dx/dt"=w483:dbl)  [unwired: 1 in, 1 out]
                      n160 = call <vilib>:"Derivative x(t) PtByPt.vi"("dt"=w477, "initial condition"=w479, "x"=w479) -> ("dx/dt"=w482:dbl)  [unwired: 1 in, 1 out]
                      n161 = call <vilib>:"Derivative x(t) PtByPt.vi"("dt"=w477, "initial condition"=w478, "x"=w478) -> ("dx/dt"=w481:dbl)  [unwired: 1 in, 1 out]
                    }
                    frame 3 {
                      n162 = call <vilib>:"Derivative x(t) PtByPt.vi"("dt"=w484, "initial condition"=w487, "x"=w487) -> ("dx/dt"=w490:dbl)  [unwired: 1 in, 1 out]
                      n163 = call <vilib>:"Derivative x(t) PtByPt.vi"("dt"=w484, "initial condition"=w486, "x"=w486) -> ("dx/dt"=w489:dbl)  [unwired: 1 in, 1 out]
                      n164 = call <vilib>:"Derivative x(t) PtByPt.vi"("dt"=w484, "initial condition"=w485, "x"=w485) -> ("dx/dt"=w488:dbl)  [unwired: 1 in, 1 out]
                    }
                    frame 4 {
                      n165 = call <vilib>:"Derivative x(t) PtByPt.vi"("dt"=w491, "initial condition"=w494, "x"=w494) -> ("dx/dt"=w497:dbl)  [unwired: 1 in, 1 out]
                      n166 = call <vilib>:"Derivative x(t) PtByPt.vi"("dt"=w491, "initial condition"=w493, "x"=w493) -> ("dx/dt"=w496:dbl)  [unwired: 1 in, 1 out]
                      n167 = call <vilib>:"Derivative x(t) PtByPt.vi"("dt"=w491, "initial condition"=w492, "x"=w492) -> ("dx/dt"=w495:dbl)  [unwired: 1 in, 1 out]
                    }
                    frame 5 {
                      n168 = call <vilib>:"Derivative x(t) PtByPt.vi"("dt"=w498, "initial condition"=w501, "x"=w501) -> ("dx/dt"=w504:dbl)  [unwired: 1 in, 1 out]
                      n169 = call <vilib>:"Derivative x(t) PtByPt.vi"("dt"=w498, "initial condition"=w500, "x"=w500) -> ("dx/dt"=w503:dbl)  [unwired: 1 in, 1 out]
                      n170 = call <vilib>:"Derivative x(t) PtByPt.vi"("dt"=w498, "initial condition"=w499, "x"=w499) -> ("dx/dt"=w502:dbl)  [unwired: 1 in, 1 out]
                    }
                  }
                  n171 = Build Array(w450, w459, w454, w458, w453, w457) -> (w456:dbl[])
                  n172 = call-poly <vilib>:"Array To Matrix.vi"("Real 1D Array"=w456) -> ("Real Matrix (Column Vector)"=w455:T4)
                  n173 = Bundle By Name(cluster=w460, "x_k|k"=w455) -> (w451:T3)
                }
              }
              frame True {
              }
            }
            n174 = case shown="False" w363 {
              tunnel: w362 -> [w373 w387]
              tunnel: w361 -> [w374 _]
              tunnel: [w372 w387] -> w360
              frame False {
                n175 = for {
                  tunnel: w373 -> [w386] mode=indexing
                  tunnel: w374 -> [w375]
                  tunnel: w373 -> [w385] mode=indexing
                  tunnel: [w376] -> w372 mode=indexing
                  n176 = Unbundle By Name(w386) -> ("x"=w380:sgl, "y"=w379:sgl, "z"=w381:sgl)
                  n177 = call <vilib>:"Derivative x(t) PtByPt.vi"("dt"=w375, "initial condition"=w380, "x"=w380) -> ("dx/dt"=w384:dbl)  [unwired: 1 in, 1 out]
                  n178 = call <vilib>:"Derivative x(t) PtByPt.vi"("dt"=w375, "initial condition"=w379, "x"=w379) -> ("dx/dt"=w383:dbl)  [unwired: 1 in, 1 out]
                  n179 = call <vilib>:"Derivative x(t) PtByPt.vi"("dt"=w375, "initial condition"=w381, "x"=w381) -> ("dx/dt"=w382:dbl)  [unwired: 1 in, 1 out]
                  n180 = Build Array(w380, w384, w379, w383, w381, w382) -> (w378:dbl[])
                  n181 = call-poly <vilib>:"Array To Matrix.vi"("Real 1D Array"=w378) -> ("Real Matrix (Column Vector)"=w377:T4)
                  n182 = Bundle By Name(cluster=w385, "x_k|k"=w377) -> (w376:T5)
                }
              }
              frame True {
              }
            }
            n183 = case shown="False" w368 {
              tunnel: w367 -> [w389 w446]
              tunnel: w361 -> [w390 _]
              tunnel: [w388 w446] -> w365
              frame False {
                n184 = for {
                  tunnel: w389 -> [w403] mode=indexing
                  tunnel: w390 -> [w391]
                  tunnel: w389 -> [w401] mode=indexing
                  tunnel: [w392] -> w388 mode=indexing
                  n185 = Unbundle By Name(w403) -> ("x"=w396:sgl, "y"=w395:sgl, "orientation"=w397:sgl, "robot_id"=w402:u32)
                  n186 = case shown="0, Default" w402 {
                    tunnel: w396 -> [w407 w414 w421 w428 w435 w442]
                    tunnel: w395 -> [w405 w412 w419 w426 w433 w440]
                    tunnel: w397 -> [w404 w411 w418 w425 w432 w439]
                    tunnel: [w410 w417 w424 w431 w438 w445] -> w400
                    tunnel: [w409 w416 w423 w430 w437 w444] -> w399
                    tunnel: [w408 w415 w422 w429 w436 w443] -> w398
                    tunnel: w391 -> [w406 w413 w420 w427 w434 w441]
                    frame 0, Default {
                      n187 = call <vilib>:"Derivative x(t) PtByPt.vi"("dt"=w406, "initial condition"=w407, "x"=w407) -> ("dx/dt"=w410:dbl)  [unwired: 1 in, 1 out]
                      n188 = call <vilib>:"Derivative x(t) PtByPt.vi"("dt"=w406, "initial condition"=w405, "x"=w405) -> ("dx/dt"=w409:dbl)  [unwired: 1 in, 1 out]
                      n189 = call <vilib>:"Derivative x(t) PtByPt.vi"("dt"=w406, "initial condition"=w404, "x"=w404) -> ("dx/dt"=w408:dbl)  [unwired: 1 in, 1 out]
                    }
                    frame 1 {
                      n190 = call <vilib>:"Derivative x(t) PtByPt.vi"("dt"=w413, "initial condition"=w414, "x"=w414) -> ("dx/dt"=w417:dbl)  [unwired: 1 in, 1 out]
                      n191 = call <vilib>:"Derivative x(t) PtByPt.vi"("dt"=w413, "initial condition"=w412, "x"=w412) -> ("dx/dt"=w416:dbl)  [unwired: 1 in, 1 out]
                      n192 = call <vilib>:"Derivative x(t) PtByPt.vi"("dt"=w413, "initial condition"=w411, "x"=w411) -> ("dx/dt"=w415:dbl)  [unwired: 1 in, 1 out]
                    }
                    frame 2 {
                      n193 = call <vilib>:"Derivative x(t) PtByPt.vi"("dt"=w420, "initial condition"=w421, "x"=w421) -> ("dx/dt"=w424:dbl)  [unwired: 1 in, 1 out]
                      n194 = call <vilib>:"Derivative x(t) PtByPt.vi"("dt"=w420, "initial condition"=w419, "x"=w419) -> ("dx/dt"=w423:dbl)  [unwired: 1 in, 1 out]
                      n195 = call <vilib>:"Derivative x(t) PtByPt.vi"("dt"=w420, "initial condition"=w418, "x"=w418) -> ("dx/dt"=w422:dbl)  [unwired: 1 in, 1 out]
                    }
                    frame 3 {
                      n196 = call <vilib>:"Derivative x(t) PtByPt.vi"("dt"=w427, "initial condition"=w428, "x"=w428) -> ("dx/dt"=w431:dbl)  [unwired: 1 in, 1 out]
                      n197 = call <vilib>:"Derivative x(t) PtByPt.vi"("dt"=w427, "initial condition"=w426, "x"=w426) -> ("dx/dt"=w430:dbl)  [unwired: 1 in, 1 out]
                      n198 = call <vilib>:"Derivative x(t) PtByPt.vi"("dt"=w427, "initial condition"=w425, "x"=w425) -> ("dx/dt"=w429:dbl)  [unwired: 1 in, 1 out]
                    }
                    frame 4 {
                      n199 = call <vilib>:"Derivative x(t) PtByPt.vi"("dt"=w434, "initial condition"=w435, "x"=w435) -> ("dx/dt"=w438:dbl)  [unwired: 1 in, 1 out]
                      n200 = call <vilib>:"Derivative x(t) PtByPt.vi"("dt"=w434, "initial condition"=w433, "x"=w433) -> ("dx/dt"=w437:dbl)  [unwired: 1 in, 1 out]
                      n201 = call <vilib>:"Derivative x(t) PtByPt.vi"("dt"=w434, "initial condition"=w432, "x"=w432) -> ("dx/dt"=w436:dbl)  [unwired: 1 in, 1 out]
                    }
                    frame 5 {
                      n202 = call <vilib>:"Derivative x(t) PtByPt.vi"("dt"=w441, "initial condition"=w442, "x"=w442) -> ("dx/dt"=w445:dbl)  [unwired: 1 in, 1 out]
                      n203 = call <vilib>:"Derivative x(t) PtByPt.vi"("dt"=w441, "initial condition"=w440, "x"=w440) -> ("dx/dt"=w444:dbl)  [unwired: 1 in, 1 out]
                      n204 = call <vilib>:"Derivative x(t) PtByPt.vi"("dt"=w441, "initial condition"=w439, "x"=w439) -> ("dx/dt"=w443:dbl)  [unwired: 1 in, 1 out]
                    }
                  }
                  n205 = Build Array(w396, w400, w395, w399, w397, w398) -> (w394:dbl[])
                  n206 = call-poly <vilib>:"Array To Matrix.vi"("Real 1D Array"=w394) -> ("Real Matrix (Column Vector)"=w393:T4)
                  n207 = Bundle By Name(cluster=w401, "x_k|k"=w393) -> (w392:T3)
                }
              }
              frame True {
              }
            }
            n208 = Bundle By Name(cluster=w359, "robots_blue"=w366, "robots_yellow"=w365, "balls"=w360) -> (w364:T2)
          }
          frame 3 {
            n209 = Empty Array?(array=w509) -> (empty?=w510:bool)
            n210 = Empty Array?(array=w514) -> (empty?=w515:bool)
            n211 = Reciprocal(x=w516) -> (1/x=w508:dbl)
            n212 = Empty Array?(array=w517) -> (empty?=w518:bool)
            n213 = case shown="False" w518 {
              tunnel: w517 -> [w595 w652]
              tunnel: w508 -> [w596 _]
              tunnel: [w594 w652] -> w513
              frame False {
                n214 = for {
                  tunnel: w595 -> [w609] mode=indexing
                  tunnel: w596 -> [w599]
                  tunnel: w595 -> [w607] mode=indexing
                  tunnel: [w598] -> w594 mode=indexing
                  n215 = Unbundle By Name(w609) -> ("x"=w597:sgl, "y"=w601:sgl, "orientation"=w600:sgl, "robot_id"=w608:u32)
                  n216 = case shown="0, Default" w608 {
                    tunnel: w597 -> [w610 w620 w627 w634 w641 w648]
                    tunnel: [w616 w623 w630 w637 w644 w651] -> w606
                    tunnel: [w615 w622 w629 w636 w643 w650] -> w605
                    tunnel: [w614 w621 w628 w635 w642 w649] -> w604
                    tunnel: w601 -> [w613 w619 w626 w633 w640 w647]
                    tunnel: w600 -> [w612 w618 w625 w632 w639 w646]
                    tunnel: w599 -> [w611 w617 w624 w631 w638 w645]
                    frame 0, Default {
                      n217 = call <vilib>:"Derivative x(t) PtByPt.vi"("dt"=w611, "initial condition"=w610, "x"=w610) -> ("dx/dt"=w616:dbl)  [unwired: 1 in, 1 out]
                      n218 = call <vilib>:"Derivative x(t) PtByPt.vi"("dt"=w611, "initial condition"=w613, "x"=w613) -> ("dx/dt"=w615:dbl)  [unwired: 1 in, 1 out]
                      n219 = call <vilib>:"Derivative x(t) PtByPt.vi"("dt"=w611, "initial condition"=w612, "x"=w612) -> ("dx/dt"=w614:dbl)  [unwired: 1 in, 1 out]
                    }
                    frame 1 {
                      n220 = call <vilib>:"Derivative x(t) PtByPt.vi"("dt"=w617, "initial condition"=w620, "x"=w620) -> ("dx/dt"=w623:dbl)  [unwired: 1 in, 1 out]
                      n221 = call <vilib>:"Derivative x(t) PtByPt.vi"("dt"=w617, "initial condition"=w619, "x"=w619) -> ("dx/dt"=w622:dbl)  [unwired: 1 in, 1 out]
                      n222 = call <vilib>:"Derivative x(t) PtByPt.vi"("dt"=w617, "initial condition"=w618, "x"=w618) -> ("dx/dt"=w621:dbl)  [unwired: 1 in, 1 out]
                    }
                    frame 2 {
                      n223 = call <vilib>:"Derivative x(t) PtByPt.vi"("dt"=w624, "initial condition"=w627, "x"=w627) -> ("dx/dt"=w630:dbl)  [unwired: 1 in, 1 out]
                      n224 = call <vilib>:"Derivative x(t) PtByPt.vi"("dt"=w624, "initial condition"=w626, "x"=w626) -> ("dx/dt"=w629:dbl)  [unwired: 1 in, 1 out]
                      n225 = call <vilib>:"Derivative x(t) PtByPt.vi"("dt"=w624, "initial condition"=w625, "x"=w625) -> ("dx/dt"=w628:dbl)  [unwired: 1 in, 1 out]
                    }
                    frame 3 {
                      n226 = call <vilib>:"Derivative x(t) PtByPt.vi"("dt"=w631, "initial condition"=w634, "x"=w634) -> ("dx/dt"=w637:dbl)  [unwired: 1 in, 1 out]
                      n227 = call <vilib>:"Derivative x(t) PtByPt.vi"("dt"=w631, "initial condition"=w633, "x"=w633) -> ("dx/dt"=w636:dbl)  [unwired: 1 in, 1 out]
                      n228 = call <vilib>:"Derivative x(t) PtByPt.vi"("dt"=w631, "initial condition"=w632, "x"=w632) -> ("dx/dt"=w635:dbl)  [unwired: 1 in, 1 out]
                    }
                    frame 4 {
                      n229 = call <vilib>:"Derivative x(t) PtByPt.vi"("dt"=w638, "initial condition"=w641, "x"=w641) -> ("dx/dt"=w644:dbl)  [unwired: 1 in, 1 out]
                      n230 = call <vilib>:"Derivative x(t) PtByPt.vi"("dt"=w638, "initial condition"=w640, "x"=w640) -> ("dx/dt"=w643:dbl)  [unwired: 1 in, 1 out]
                      n231 = call <vilib>:"Derivative x(t) PtByPt.vi"("dt"=w638, "initial condition"=w639, "x"=w639) -> ("dx/dt"=w642:dbl)  [unwired: 1 in, 1 out]
                    }
                    frame 5 {
                      n232 = call <vilib>:"Derivative x(t) PtByPt.vi"("dt"=w645, "initial condition"=w648, "x"=w648) -> ("dx/dt"=w651:dbl)  [unwired: 1 in, 1 out]
                      n233 = call <vilib>:"Derivative x(t) PtByPt.vi"("dt"=w645, "initial condition"=w647, "x"=w647) -> ("dx/dt"=w650:dbl)  [unwired: 1 in, 1 out]
                      n234 = call <vilib>:"Derivative x(t) PtByPt.vi"("dt"=w645, "initial condition"=w646, "x"=w646) -> ("dx/dt"=w649:dbl)  [unwired: 1 in, 1 out]
                    }
                  }
                  n235 = Build Array(w597, w606, w601, w605, w600, w604) -> (w603:dbl[])
                  n236 = call-poly <vilib>:"Array To Matrix.vi"("Real 1D Array"=w603) -> ("Real Matrix (Column Vector)"=w602:T4)
                  n237 = Bundle By Name(cluster=w607, "x_k|k"=w602) -> (w598:T3)
                }
              }
              frame True {
              }
            }
            n238 = case shown="False" w510 {
              tunnel: w509 -> [w520 w534]
              tunnel: w508 -> [w521 _]
              tunnel: [w519 w534] -> w507
              frame False {
                n239 = for {
                  tunnel: w520 -> [w533] mode=indexing
                  tunnel: w521 -> [w522]
                  tunnel: w520 -> [w532] mode=indexing
                  tunnel: [w523] -> w519 mode=indexing
                  n240 = Unbundle By Name(w533) -> ("x"=w527:sgl, "y"=w526:sgl, "z"=w528:sgl)
                  n241 = call <vilib>:"Derivative x(t) PtByPt.vi"("dt"=w522, "initial condition"=w527, "x"=w527) -> ("dx/dt"=w531:dbl)  [unwired: 1 in, 1 out]
                  n242 = call <vilib>:"Derivative x(t) PtByPt.vi"("dt"=w522, "initial condition"=w526, "x"=w526) -> ("dx/dt"=w530:dbl)  [unwired: 1 in, 1 out]
                  n243 = call <vilib>:"Derivative x(t) PtByPt.vi"("dt"=w522, "initial condition"=w528, "x"=w528) -> ("dx/dt"=w529:dbl)  [unwired: 1 in, 1 out]
                  n244 = Build Array(w527, w531, w526, w530, w528, w529) -> (w525:dbl[])
                  n245 = call-poly <vilib>:"Array To Matrix.vi"("Real 1D Array"=w525) -> ("Real Matrix (Column Vector)"=w524:T4)
                  n246 = Bundle By Name(cluster=w532, "x_k|k"=w524) -> (w523:T5)
                }
              }
              frame True {
              }
            }
            n247 = case shown="False" w515 {
              tunnel: w514 -> [w536 w593]
              tunnel: w508 -> [w537 _]
              tunnel: [w535 w593] -> w512
              frame False {
                n248 = for {
                  tunnel: w536 -> [w550] mode=indexing
                  tunnel: w537 -> [w538]
                  tunnel: w536 -> [w548] mode=indexing
                  tunnel: [w539] -> w535 mode=indexing
                  n249 = Unbundle By Name(w550) -> ("x"=w543:sgl, "y"=w542:sgl, "orientation"=w544:sgl, "robot_id"=w549:u32)
                  n250 = case shown="0, Default" w549 {
                    tunnel: w543 -> [w554 w561 w568 w575 w582 w589]
                    tunnel: w542 -> [w552 w559 w566 w573 w580 w587]
                    tunnel: w544 -> [w551 w558 w565 w572 w579 w586]
                    tunnel: [w557 w564 w571 w578 w585 w592] -> w547
                    tunnel: [w556 w563 w570 w577 w584 w591] -> w546
                    tunnel: [w555 w562 w569 w576 w583 w590] -> w545
                    tunnel: w538 -> [w553 w560 w567 w574 w581 w588]
                    frame 0, Default {
                      n251 = call <vilib>:"Derivative x(t) PtByPt.vi"("dt"=w553, "initial condition"=w554, "x"=w554) -> ("dx/dt"=w557:dbl)  [unwired: 1 in, 1 out]
                      n252 = call <vilib>:"Derivative x(t) PtByPt.vi"("dt"=w553, "initial condition"=w552, "x"=w552) -> ("dx/dt"=w556:dbl)  [unwired: 1 in, 1 out]
                      n253 = call <vilib>:"Derivative x(t) PtByPt.vi"("dt"=w553, "initial condition"=w551, "x"=w551) -> ("dx/dt"=w555:dbl)  [unwired: 1 in, 1 out]
                    }
                    frame 1 {
                      n254 = call <vilib>:"Derivative x(t) PtByPt.vi"("dt"=w560, "initial condition"=w561, "x"=w561) -> ("dx/dt"=w564:dbl)  [unwired: 1 in, 1 out]
                      n255 = call <vilib>:"Derivative x(t) PtByPt.vi"("dt"=w560, "initial condition"=w559, "x"=w559) -> ("dx/dt"=w563:dbl)  [unwired: 1 in, 1 out]
                      n256 = call <vilib>:"Derivative x(t) PtByPt.vi"("dt"=w560, "initial condition"=w558, "x"=w558) -> ("dx/dt"=w562:dbl)  [unwired: 1 in, 1 out]
                    }
                    frame 2 {
                      n257 = call <vilib>:"Derivative x(t) PtByPt.vi"("dt"=w567, "initial condition"=w568, "x"=w568) -> ("dx/dt"=w571:dbl)  [unwired: 1 in, 1 out]
                      n258 = call <vilib>:"Derivative x(t) PtByPt.vi"("dt"=w567, "initial condition"=w566, "x"=w566) -> ("dx/dt"=w570:dbl)  [unwired: 1 in, 1 out]
                      n259 = call <vilib>:"Derivative x(t) PtByPt.vi"("dt"=w567, "initial condition"=w565, "x"=w565) -> ("dx/dt"=w569:dbl)  [unwired: 1 in, 1 out]
                    }
                    frame 3 {
                      n260 = call <vilib>:"Derivative x(t) PtByPt.vi"("dt"=w574, "initial condition"=w575, "x"=w575) -> ("dx/dt"=w578:dbl)  [unwired: 1 in, 1 out]
                      n261 = call <vilib>:"Derivative x(t) PtByPt.vi"("dt"=w574, "initial condition"=w573, "x"=w573) -> ("dx/dt"=w577:dbl)  [unwired: 1 in, 1 out]
                      n262 = call <vilib>:"Derivative x(t) PtByPt.vi"("dt"=w574, "initial condition"=w572, "x"=w572) -> ("dx/dt"=w576:dbl)  [unwired: 1 in, 1 out]
                    }
                    frame 4 {
                      n263 = call <vilib>:"Derivative x(t) PtByPt.vi"("dt"=w581, "initial condition"=w582, "x"=w582) -> ("dx/dt"=w585:dbl)  [unwired: 1 in, 1 out]
                      n264 = call <vilib>:"Derivative x(t) PtByPt.vi"("dt"=w581, "initial condition"=w580, "x"=w580) -> ("dx/dt"=w584:dbl)  [unwired: 1 in, 1 out]
                      n265 = call <vilib>:"Derivative x(t) PtByPt.vi"("dt"=w581, "initial condition"=w579, "x"=w579) -> ("dx/dt"=w583:dbl)  [unwired: 1 in, 1 out]
                    }
                    frame 5 {
                      n266 = call <vilib>:"Derivative x(t) PtByPt.vi"("dt"=w588, "initial condition"=w589, "x"=w589) -> ("dx/dt"=w592:dbl)  [unwired: 1 in, 1 out]
                      n267 = call <vilib>:"Derivative x(t) PtByPt.vi"("dt"=w588, "initial condition"=w587, "x"=w587) -> ("dx/dt"=w591:dbl)  [unwired: 1 in, 1 out]
                      n268 = call <vilib>:"Derivative x(t) PtByPt.vi"("dt"=w588, "initial condition"=w586, "x"=w586) -> ("dx/dt"=w590:dbl)  [unwired: 1 in, 1 out]
                    }
                  }
                  n269 = Build Array(w543, w547, w542, w546, w544, w545) -> (w541:dbl[])
                  n270 = call-poly <vilib>:"Array To Matrix.vi"("Real 1D Array"=w541) -> ("Real Matrix (Column Vector)"=w540:T4)
                  n271 = Bundle By Name(cluster=w548, "x_k|k"=w540) -> (w539:T3)
                }
              }
              frame True {
              }
            }
            n272 = Bundle By Name(cluster=w506, "robots_blue"=w513, "robots_yellow"=w512, "balls"=w507) -> (w511:T2)
          }
        }
      }
      frame "Nenhum" {
      }
    }
  }
  n273 = feedback-in #1(w26) -> ()
  n274 = feedback-in #3(w15) -> ()
  n275 = disable-structure shown="Enabled" {
    disable-tunnel: _ -> [w667 _]
    disable-tunnel: _ -> [w666 _]
    disable-tunnel: _ -> [w665 _]
    disable-tunnel: _ -> [w660 _]
    disable-tunnel: w15 -> [w657 w671]
    disable-tunnel: [_ w670] -> w3
    disable-tunnel: "cameras array" -> [_ w669]
    disable-tunnel: "grSim?" -> [_ w668]
    disable-tunnel: "Field" -> [_ _]
    frame Disabled {
      n276 = Bundle By Name(cluster=w667, "robots_yellow"=w666, "robots_blue"=w665, "balls"=w660) -> (w656:cluster{})
      n277 = Unbundle By Name(w656) -> ("balls"=w659, "robots_yellow"=w662, "robots_blue"=w664)
      n278 = call "Select Robots By Confidence.vi"("robots_blue"=w662) -> ("Array"=w661:T3[])  [unwired: 10 in]
      n279 = call "Select Ball By Confidence.vi"("Array"=w657, "balls"=w659) -> ("balls out"=w658:T5[])  [unwired: 9 in]
      n280 = call "Select Robots By Confidence.vi"("robots_blue"=w664) -> ("Array"=w663:T3[])  [unwired: 10 in]
      n281 = Bundle By Name(cluster=w656, "balls"=w658, "robots_yellow"=w661, "robots_blue"=w663) -> (w655:cluster{})
    }
    frame Enabled {
      n282 = call "mediaIntesecaoCameras_v2.vi"("grsim?"=w668, "cameras array"=w669, "Cameras Array"=w671) -> ("frame out"=w670:T2)  [unwired: 8 in]
    }
  }
  n283 = Unbundle By Name(w3) -> ("balls"=w8:T5[], "robots_blue"=w7:T3[], "robots_yellow"=w4:T3[])
  n284 = feedback-in #2(w8) -> ()
  n285 = feedback #4(w7) -> (w9:T3[])
  n286 = call "NewLifetimeForRobot.vi"("Last robots"=w9, "Current robots"=w7) -> ("Array of robots"=w10:T3[])  [unwired: 9 in]
  n287 = feedback-in #4(w10) -> ()
  n288 = feedback #5(w8) -> (w11:T5[])
  n289 = call "NewBallLifetime.vi"("last balls"=w11, "current ball"=w8) -> ("balls out"=w12:T5[])  [unwired: 9 in]
  n290 = feedback-in #5(w12) -> ()
  n291 = feedback #6(w4) -> (w5:T3[])
  n292 = call "NewLifetimeForRobot.vi"("Last robots"=w5, "Current robots"=w4) -> ("Array of robots"=w6:T3[])  [unwired: 9 in]
  n293 = feedback-in #6(w6) -> ()
  n294 = Bundle By Name(cluster=w3, "balls"=w12, "robots_blue"=w10, "robots_yellow"=w6) -> (→"Detection Frame Out":T2)
  "Field" <- "Field"
